vi "IntakeManual.vi"() -> (2 "RollerSpeed":dbl, 3 "ArmSpeed":dbl)   [LabVIEW 2015]
uses:
  Robot Global Data.vi
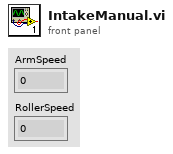
[diagram p1: front panel]
types:
  T1 = typedef "IntakeManual.ctl" = cluster{"RollerSpeed":dbl, "ArmSpeed":dbl, "ManualCommand":enum16{"Idle", "BallIn", "BallOut", "ArmUp", "ArmDown"}}
  T2 = enum16{"Idle", "BallIn", "BallOut", "ArmUp", "ArmDown"}
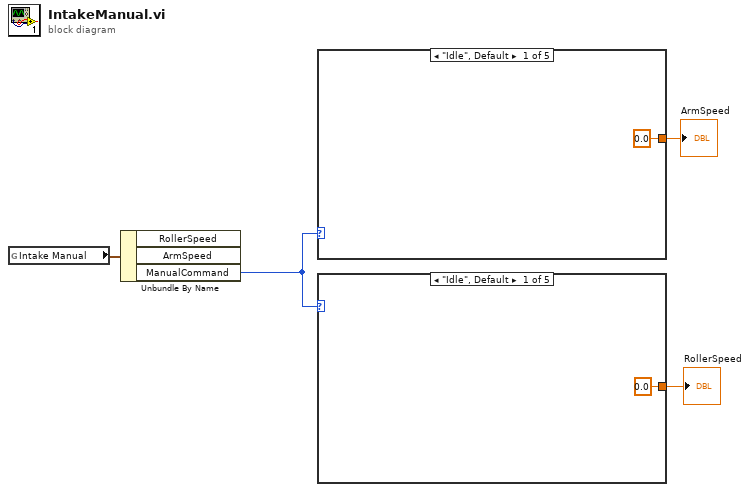
[diagram p0: block diagram]
diagram:
  n1 = global read "Robot Global Data.vi" "Intake Manual"() -> (w4:T1)
  n2 = Unbundle By Name(w4) -> ("ManualCommand"=w3:T2)  [unwired: 2 out]
  n3 = case shown="\"Idle\", Default" w3 {
    tunnel: [0.0 _ _ _ _] -> w1
    frame "Idle", Default {
    }
    frame "BallIn" {
    }
    frame "BallOut" {
    }
    frame "ArmUp" {
    }
    frame "ArmDown" {
    }
  }
  "ArmSpeed" <- w1
  n4 = case shown="\"Idle\", Default" w3 {
    tunnel: [0.0 _ _ _ _] -> w2
    frame "Idle", Default {
    }
    frame "BallIn" {
    }
    frame "BallOut" {
    }
    frame "ArmUp" {
    }
    frame "ArmDown" {
    }
  }
  "RollerSpeed" <- w2
